vi "RC_PWM_to_01.vi"(8 "error in (no error)":errorcluster, 11 "Refnum in":refnum<k20>) -> (0 "error out":errorcluster, 1 "Use RC Control?":bool, 2 "Rudder Control Output":dbl, 3 "Hand Sail Control":T1 {"MainSailSuggestion" min=0.0 max=1.0; "JibSailSuggestion" min=0.0 max=1.0}, 4 "Sail Debug Output":dbl)   [LabVIEW 2013]
doc: "This VI takes the PWM read FPGA code and reads values from the controller. We determined via testing the constants that let us take PWM values and convert them to 0,1 for the sails and -1,1 for the sails.\n\nThere is jitter detection in this code. If the command value changed by less than 0.03 from the last command, then the command is unchanged from before. This removes a constant small jitter from the read PWM value.\n\nEric Schneider, December 2014"
uses:
  Data/TypeDefs/Sail Set Suggestions.ctl
  <vilib>/rvi/interface/common/niFpgaWaitOnOcc.vi
  <vilib>/Utility/error.llb/Error Cluster From Error Code.vi
  <vilib>/rvi/errors/niLvFpgaAdjustHostInterfaceError.vi
  <vilib>/rvi/interface/nirviReadWriteControl/nirviReadWriteControl.xnode
  NiFpgaLv.dll
  <vilib>/rvi/interface/Simulation/niFpgaSimulationCallBeginRW.vi
panel:
  in  "RC/Autonomous Control Switch Threshold":dbl=0.065
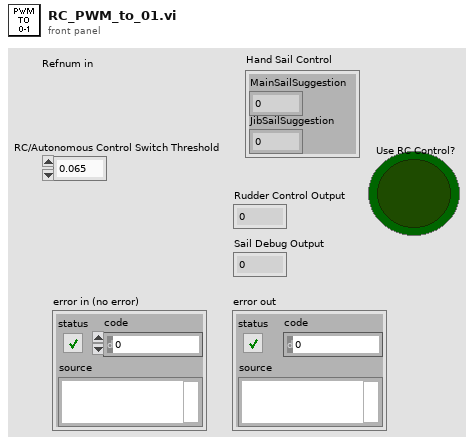
[diagram p1: front panel]
types:
  T1 = typedef "Sail Set Suggestions.ctl" = cluster{"MainSailSuggestion":dbl, "JibSailSuggestion":dbl}
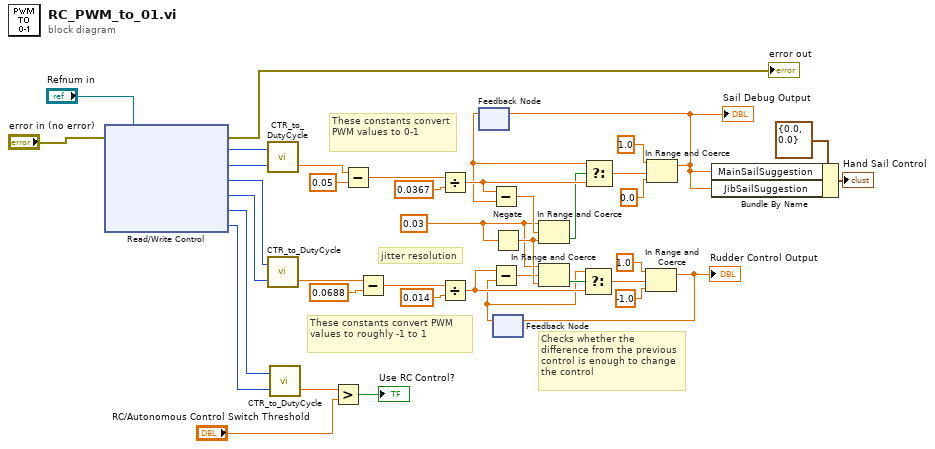
[diagram p0: block diagram]
diagram:
  w14 = 0.03 ("Jitter cutout")
  # "These constants convert PWM values to roughly -1 to 1"
  # "These constants convert PWM values to 0-1"
  # "Checks whether the difference from the previous control is enough to change the control"
  # "jitter resolution"
  n1 = xnode "Read/Write Control"("FPGA VI Reference In"="Refnum in", "error in"="error in (no error)") -> ("error out"=→"error out":errorcluster, "Sail High Center"=w21:u32, "Sail Low Center"=w22:u32, "Rudder High Center"=w23:u32, "Rudder Low Center"=w24:u32, "Switch High Center"=w5:u32, "Switch Low Center"=w4:u32)  [unwired: 1 out]
  n2 = call "CTR_to_DutyCycle.vi"("LOW CTR"=w22, "HIGH CTR"=w21) -> ("duty cycle fraction [0-1]"=w26:dbl)  [unwired: 1 out]
  n3 = call "CTR_to_DutyCycle.vi"("LOW CTR"=w24, "HIGH CTR"=w23) -> ("duty cycle fraction [0-1]"=w32:dbl)  [unwired: 1 out]
  n4 = call "CTR_to_DutyCycle.vi"("LOW CTR"=w4, "HIGH CTR"=w5) -> ("duty cycle fraction [0-1]"=w3:dbl)  [unwired: 1 out]
  n5 = Greater?(x=w3, y="RC/Autonomous Control Switch Threshold") -> (0:→"Use RC Control?":bool)
  n6 = Subtract(x=w26, y=0.05) -> (x-y=w27:dbl)
  n7 = Subtract(x=w32, y=0.0688) -> (x-y=w30:dbl)
  n8 = Divide(x=w27, y=0.0367) -> (x/y=w40:dbl)
  n9 = Divide(x=w30, y=0.014) -> (x/y=w37:dbl)
  n10 = feedback #1() -> (w19:dbl)  [unwired: 1 in]
  n11 = Subtract(x=w40, y=w19) -> (x-y=w33:dbl)
  n12 = Negate(x=w14) -> (-x=w39:dbl)
  n13 = feedback #2() -> (w20:dbl)  [unwired: 1 in]
  n14 = Subtract(x=w37, y=w20) -> (x-y=w35:dbl)
  n15 = In Range and Coerce(upper limit=w14, x=w33, lower limit=w39) -> (In Range?=w34:bool)  [unwired: 1 out]
  n16 = In Range and Coerce(upper limit=w14, x=w35, lower limit=w39) -> (In Range?=w36:bool)  [unwired: 1 out]
  n17 = Select(t=w20, s=w36, f=w37) -> (s? t:f=w12:dbl)
  n18 = Select(t=w19, s=w34, f=w40) -> (s? t:f=w7:dbl)
  n19 = In Range and Coerce(upper limit=1.0, x=w12, lower limit=-1.0) -> (coerced(x)=w13:dbl)  [unwired: 1 out]
  "Rudder Control Output" <- w13
  n20 = feedback-in #2(w13) -> ()
  n21 = In Range and Coerce(upper limit=1.0, x=w7, lower limit=0.0) -> (coerced(x)=w6:dbl)  [unwired: 1 out]
  "Sail Debug Output" <- w6
  n22 = feedback-in #1(w6) -> ()
  n23 = Bundle By Name(cluster=T1 {"MainSailSuggestion"=0.0, "JibSailSuggestion"=0.0} ("Hand Sail Control"), "MainSailSuggestion"=w6, "JibSailSuggestion"=w6) -> (→"Hand Sail Control":T1)
